vi "AddCount_Queue.vi"(9 "Counters Monitor Array IN":T1(array[cluster]), 11 "QueueElementIn":string) -> (1 "Counters Monitor Array OUT":T1(array[cluster]))   [LabVIEW 2017]
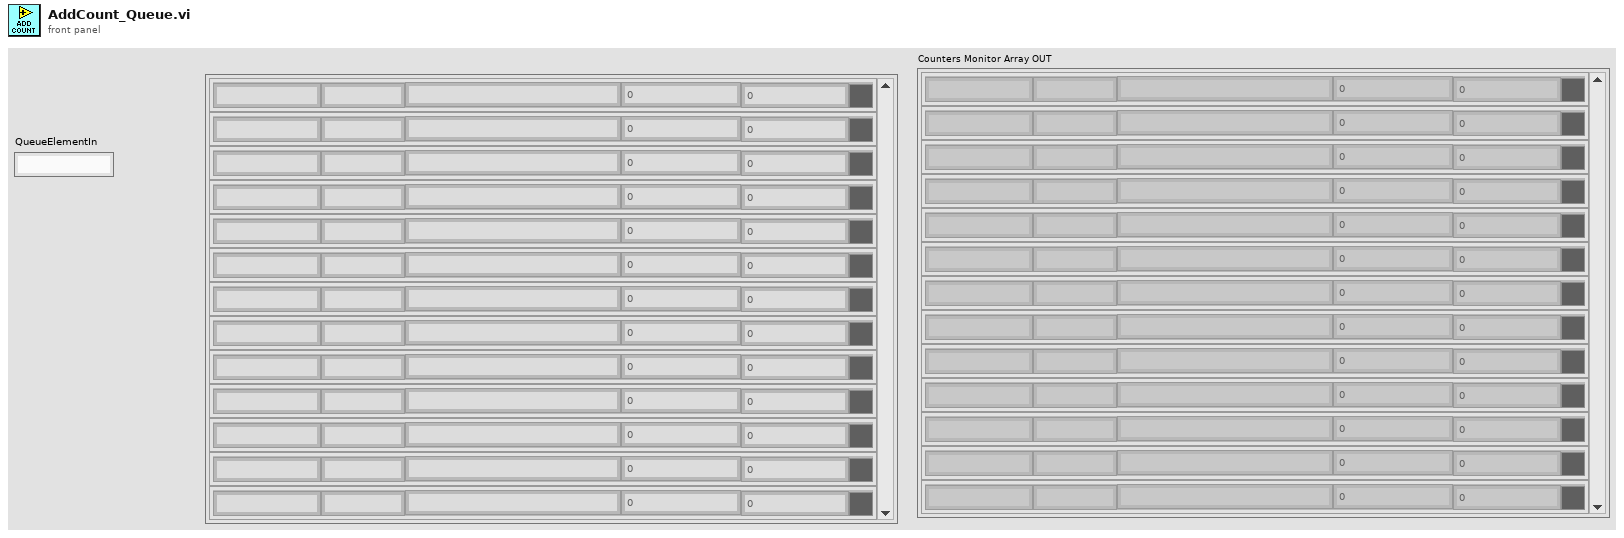
[diagram p1: front panel]
types:
  T1 = cluster{"MachineName":string, "ComponentName":string, "StoppageAlarmCounter":i32, "CurrentCount":i32, "StatusColorBox":u32, "ToolCribPartNumber":string}[]
  T2 = cluster{"MachineName":string, "ComponentName":string, "StoppageAlarmCounter":i32, "CurrentCount":i32, "StatusColorBox":u32, "ToolCribPartNumber":string}
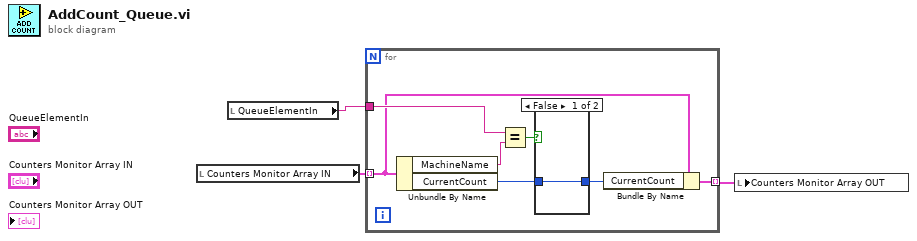
[diagram p0: block diagram]
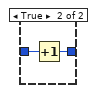
[diagram p2: hidden frame]
diagram:
  n1 = local read "Counters Monitor Array IN"() -> (w3:T1)
  n2 = local read "QueueElementIn"() -> (w1:string)
  n3 = for {
    tunnel: w3 -> [w6] mode=indexing
    tunnel: w1 -> [w9]
    tunnel: [w4] -> w2 mode=indexing
    n4 = Unbundle By Name(w6) -> ("MachineName"=w10:string, "CurrentCount"=w7:i32)
    n5 = Equal?(x=w9, y=w10) -> (x = y?=w8:bool)
    n6 = case shown="False" w8 {
      tunnel: w7 -> [w11 w13]
      tunnel: [w11 w12] -> w5
      frame False {
      }
      frame True {
        n7 = Increment(x=w13) -> (x+1=w12:i32)
      }
    }
    n8 = Bundle By Name(cluster=w6, "CurrentCount"=w5) -> (w4:T2)
  }
  n9 = local write "Counters Monitor Array OUT"(w2) -> ()
